vi "Connector2 Digital Output.vi"(0 "Packet":u64) -> ()   [LabVIEW 2010]
uses:
  <vilib>/eio/EIONode/EIONode.xnode
  <vilib>/rvi/eio/nirviEIOImplementation/nirviEIOImplementation.xnode
  <vilib>/rvi/eio/common/nirviEmuClasses.ctl
  <vilib>/rvi/eio/common/nirviEmuTemplateMethod_noerrors.vi
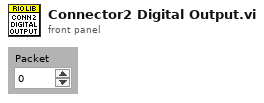
[diagram p1: front panel]
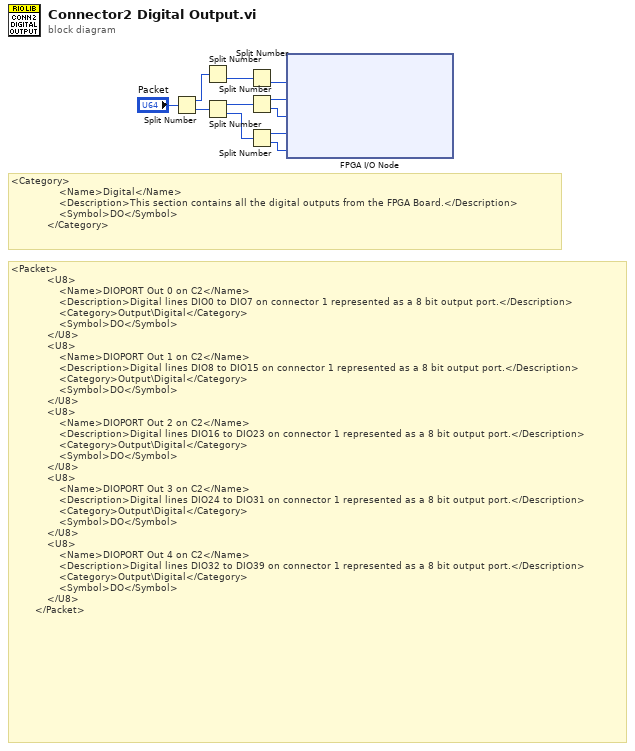
[diagram p0: block diagram]
diagram:
  # "<Category>\n                <Name>Digital</Name>\n                <Description>This section contains all the digital outputs from the FPGA Board.</Description>\n                <Symbol>DO</Symbol>\n            </Category>"
  # "<Packet>\n            <U8>\n                <Name>DIOPORT Out 0 on C2</Name>\n                <Description>Digital lines DIO0 to DIO7 on connector 1 represented as a 8 bit output port.</Description>\n                <Category>Output\\Digital</Category>\n                <Symbol>DO</Symbol>\n            </U8>\n            <U8>\n                <Name>DIOPORT Out 1 on C2</Name>\n                <Description>Digital lines DIO8 to DIO15 on connector 1 represented as a 8 bit output port.</Description>\n                <Category>Output\\Digital</Category>\n                <Symbol>DO</Symbol>\n            </U8>\n            <U8>\n                <Name>DIOPORT Out 2 on C2</Name>\n                <Description>Digital lines DIO16 to DIO23 on connector 1 represented as a 8 bit output port.</Description>\n                <Category>Output\\Digital</Category>\n                <Symbol>DO</Symbol>\n            </U8>\n            <U8>\n                <Name>DIOPORT Out 3 on C2</Name>\n                <Description>Digital lines DIO24 to DIO31 on connector 1 represented as a 8 bit output port.</Description>\n                <Category>Output\\Digital</Category>\n                <Symbol>DO</Symbol>\n            </U8>\n            <U8>\n                <Name>DIOPORT Out 4 on C2</Name>\n                <Description>Digital lines DIO32 to DIO39 on connector 1 represented as a 8 bit output port.</Description>\n                <Category>Output\\Digital</Category>\n                <Symbol>DO</Symbol>\n            </U8>\n        </Packet>"
  n1 = Split Number(x="Packet") -> (hi(x)=w7:u32, lo(x)=w6:u32)
  n2 = Split Number(x=w7) -> (lo(x)=w8:u16)  [unwired: 1 out]
  n3 = Split Number(x=w6) -> (hi(x)=w10:u16, lo(x)=w9:u16)
  n4 = Split Number(x=w8) -> (lo(x)=w1:u8)  [unwired: 1 out]
  n5 = Split Number(x=w10) -> (hi(x)=w2:u8, lo(x)=w3:u8)
  n6 = Split Number(x=w9) -> (hi(x)=w4:u8, lo(x)=w5:u8)
  n7 = xnode "FPGA I/O Node"("Connector2/DIOPORT4"=w1, "Connector2/DIOPORT3"=w2, "Connector2/DIOPORT2"=w3, "Connector2/DIOPORT1"=w4, "Connector2/DIOPORT0"=w5) -> ()  [unwired: 5 in, 5 out]
